vi "Untitled 7 (SubVI).vi"(8 "error in (no error)":errorcluster, 11 "dx":dbl) -> (0 "error out":errorcluster, 3 "out":dbl)   [LabVIEW 2023]
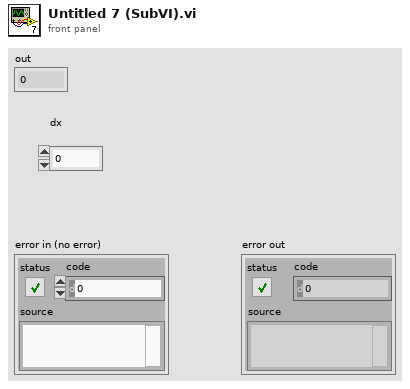
[diagram p1: front panel]
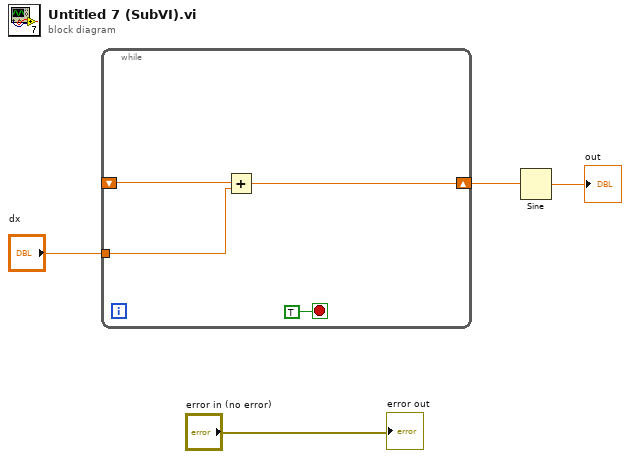
[diagram p0: block diagram]
diagram:
  n1 = while {
    shift-right: [w5] -> w1
    shift-left: _ -> [w7]
    tunnel: "dx" -> [w6]
    stop <- TRUE stop-if-true
    n2 = Add(x=w7, y=w6) -> (x+y=w5:dbl)
  }
  n3 = Sine(x=w1) -> (sin(x)=→"out":dbl)
  "error out" <- "error in (no error)"
